vi "Scripting_GetNoErrorInsideTerminals.vi"(0 "ViReference":refnum<vi>, 5 "error in (no error)":errorcluster, 6 "RemoveWire(False)":bool, 7 "OnlyTop(False)":bool, 8 "GetCaseLeftTerminals(True)":bool=TRUE) -> (13 "Bottom_InsideTermRefnumOut":refnum<vi>, 14 "Top_WireTermSource":refnum<vi>, 15 "Top_WireTermDrains":refnum<vi>[](array[refnum]), 16 "Bottom_WireTermSource":refnum<vi>, 17 "Bottom_WireTermDrains":refnum<vi>[](array[refnum]), 18 "Top_InsideTermRefnumOut":refnum<vi>, 19 "error out":errorcluster)   [LabVIEW 2020]
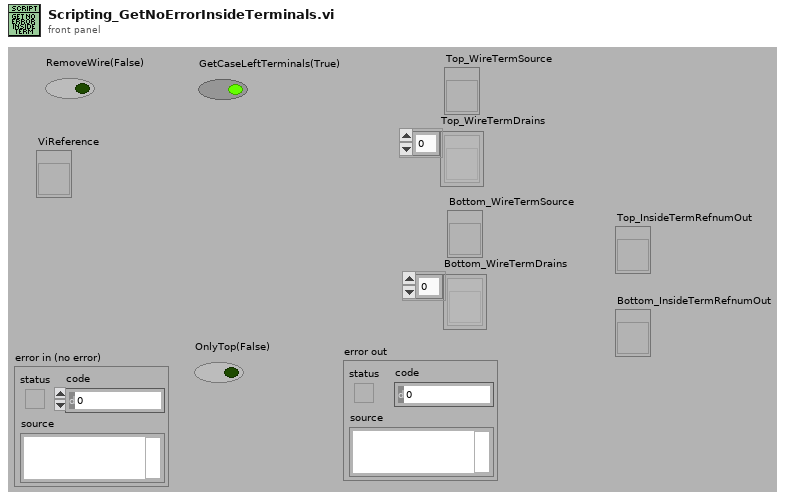
[diagram p1: front panel]
types:
  T1 = typedef "LVRectTypeDef.ctl" = cluster{"Left":i16, "Top":i16, "Right":i16, "Bottom":i16}
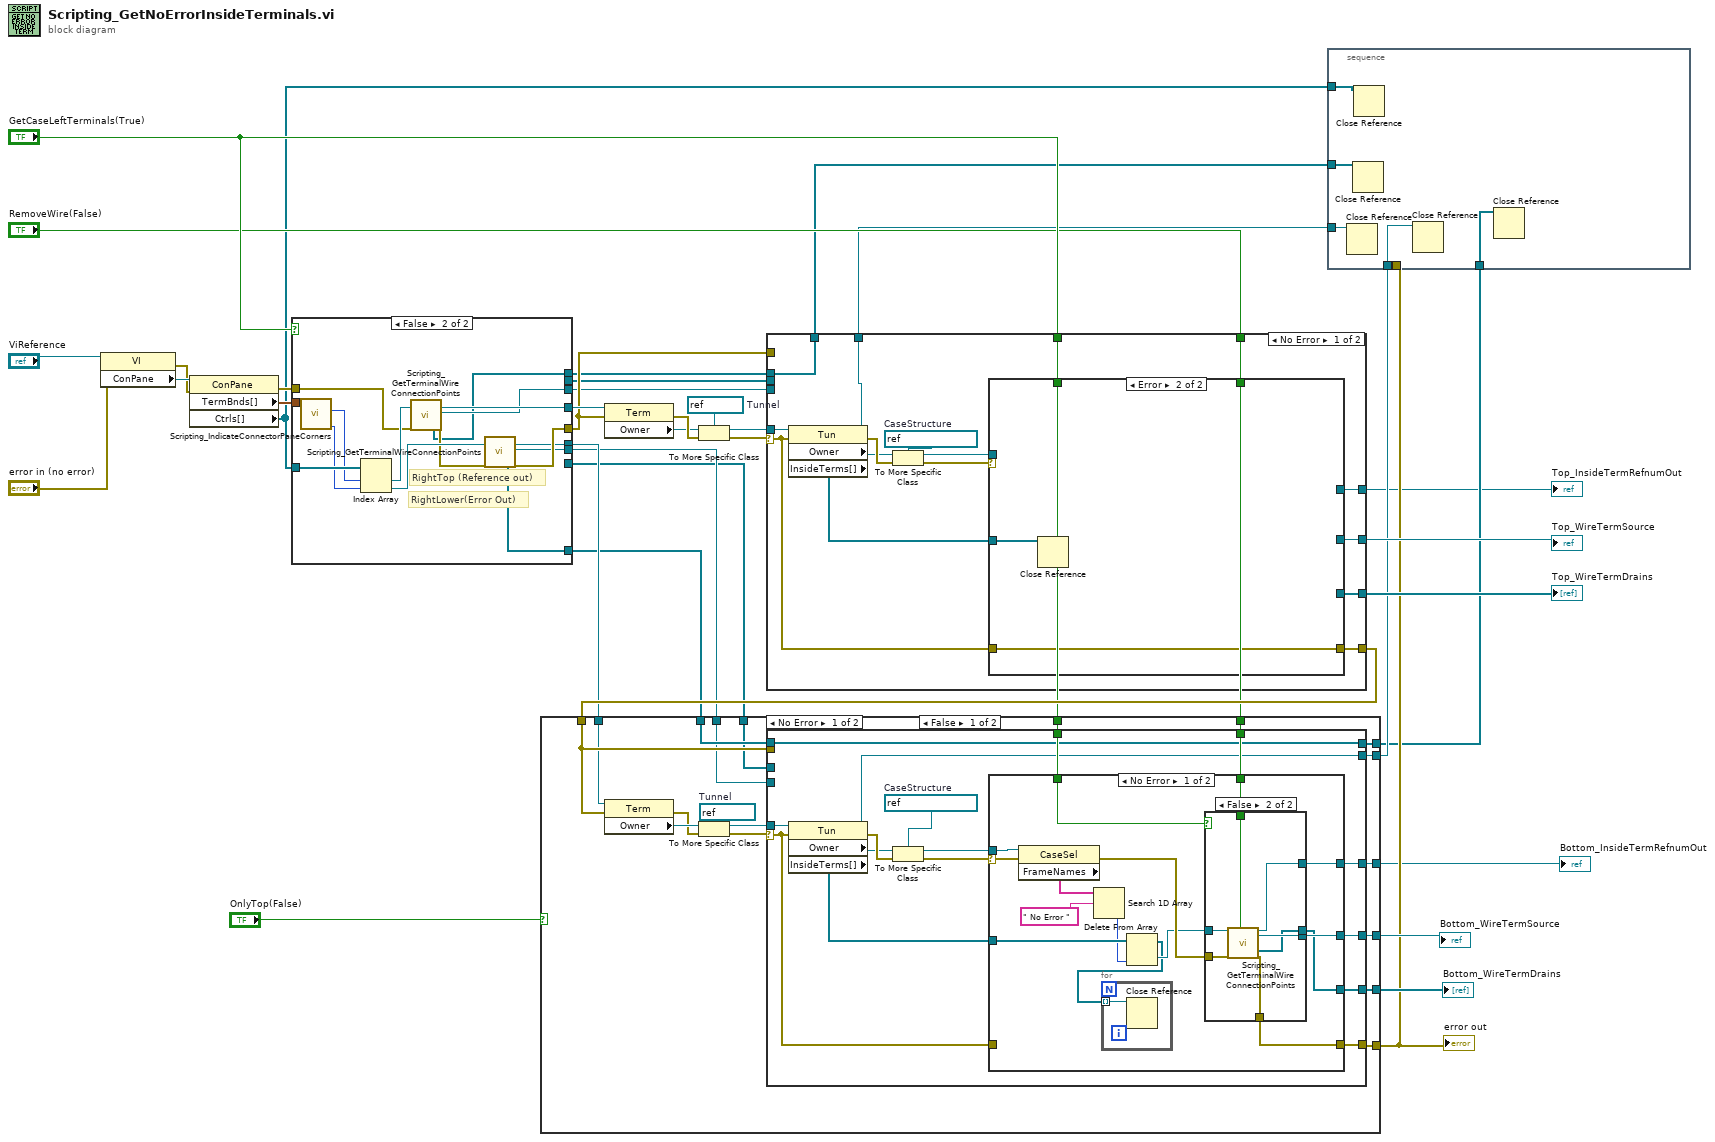
[diagram p0: block diagram]
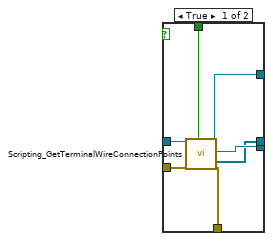
[diagram p2: hidden frame]
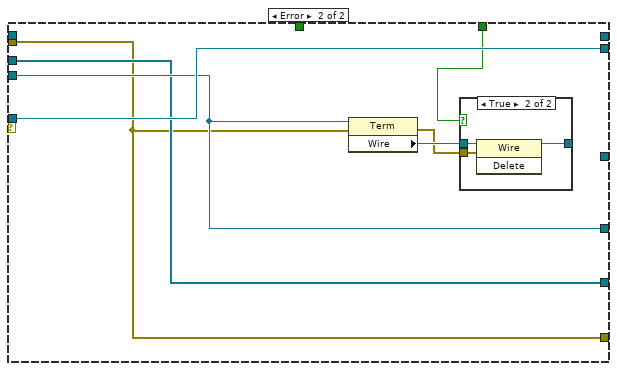
[diagram p4: hidden frame]
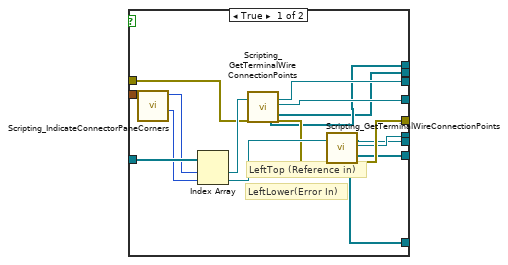
[diagram p7: hidden frame]
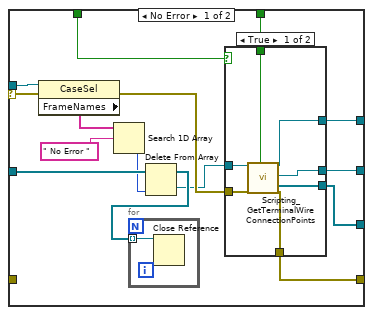
[diagram p8: hidden frame]
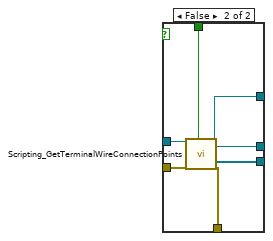
[diagram p9: hidden frame]
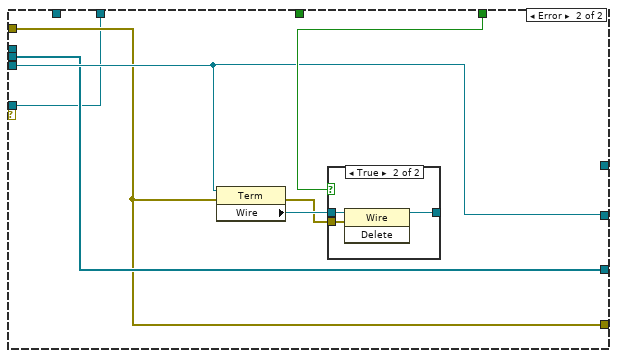
[diagram p10: hidden frame]
diagram:
  w32 = refnum<vi> refnum  # Tunnel
  n1 = property class="VI"(reference="ViReference", error in="error in (no error)") -> (error out=w23:errorcluster, "ConPane"=w35:refnum<vi>)  [unwired: 1 out]
  n2 = property class="ConPane"(reference=w35, error in=w23) -> (error out=w34:errorcluster, "TermBnds[]"=w36:T1[], "Ctrls[]"=w14:refnum<vi>[])  [unwired: 1 out]
  n3 = case shown="False" "GetCaseLeftTerminals(True)" {
    tunnel: w36 -> [w53 w68]
    tunnel: w14 -> [w52 w67]
    tunnel: w34 -> [w50 w63]
    tunnel: [w47 w62] -> w33
    tunnel: [w44 w59] -> w28
    tunnel: [w43 w58] -> w18
    tunnel: [w41 w55] -> w12
    tunnel: [w42 w57] -> w10
    tunnel: [w40 w56] -> w8
    tunnel: [w39 w54] -> w7
    tunnel: [w38 _] -> w5
    tunnel: [w37 _] -> w4
    frame True {
      # "LeftLower(Error In)"
      # "LeftTop (Reference in)"
      n4 = call "Scripting_IndicateConnectorPaneCorners.vi"("TermBnds[]"=w53) -> ("LeftLower"=w48:i32, "LeftTop"=w49:i32)  [unwired: 7 in, 2 out]
      n5 = Index Array(array=w52, index #1=w49, index #2=w48) -> (element #1=w51:refnum<vi>, element #2=w46:refnum<vi>)
      n6 = call "Scripting_GetTerminalWireConnectionPoints.vi"("ControlRef(IgnoredIfNotWired)"=w51, "error in"=w50) -> ("AllWireTerminals"=w41:refnum<vi>[], "WireTermSource"=w42:refnum<vi>, "FirstWireTermDrain"=w47:refnum<vi>, "AllWireTerminalDrains"=w37:refnum<vi>[], "error out"=w45:errorcluster)  [unwired: 9 in, 4 out]
      n7 = call "Scripting_GetTerminalWireConnectionPoints.vi"("ControlRef(IgnoredIfNotWired)"=w46, "error in"=w45) -> ("AllWireTerminals"=w40:refnum<vi>[], "WireTermSource"=w39:refnum<vi>, "FirstWireTermDrain"=w43:refnum<vi>, "AllWireTerminalDrains"=w38:refnum<vi>[], "error out"=w44:errorcluster)  [unwired: 9 in, 4 out]
    }
    frame False {
      # "RightLower(Error Out)"
      # "RightTop (Reference out)"
      n8 = call "Scripting_IndicateConnectorPaneCorners.vi"("TermBnds[]"=w68) -> ("RightLower"=w65:i32, "RightTop"=w66:i32)  [unwired: 7 in, 2 out]
      n9 = Index Array(array=w67, index #1=w66, index #2=w65) -> (element #1=w64:refnum<vi>, element #2=w61:refnum<vi>)
      n10 = call "Scripting_GetTerminalWireConnectionPoints.vi"("ControlRef(IgnoredIfNotWired)"=w64, "error in"=w63) -> ("AllWireTerminals"=w55:refnum<vi>[], "WireTermSource"=w62:refnum<vi>, "FirstWireTermDrain"=w57:refnum<vi>, "error out"=w60:errorcluster)  [unwired: 9 in, 5 out]
      n11 = call "Scripting_GetTerminalWireConnectionPoints.vi"("ControlRef(IgnoredIfNotWired)"=w61, "error in"=w60) -> ("AllWireTerminals"=w56:refnum<vi>[], "WireTermSource"=w58:refnum<vi>, "FirstWireTermDrain"=w54:refnum<vi>, "error out"=w59:errorcluster)  [unwired: 9 in, 5 out]
    }
  }
  n12 = property class="Term"(reference=w33, error in=w28) -> (error out=w31:errorcluster, "Owner"=w27:refnum<vi>)  [unwired: 1 out]
  n13 = To More Specific Class(target class=w32, reference=w27, error in=w31) -> (specific class reference=w29:refnum<vi>, error out=w30:errorcluster)
  n14 = case shown="No Error" w30 {
    selector: w30 -> [w75 _]
    tunnel: w29 -> [w84 w117]
    tunnel: w28 -> [_ w119]
    tunnel: [w78 w122] -> w26
    tunnel: [w77 w120] -> w25
    tunnel: [w76 w119] -> w21
    tunnel: "RemoveWire(False)" -> [w74 w123]
    tunnel: "GetCaseLeftTerminals(True)" -> [w72 _]
    tunnel: w12 -> [w71 _]
    tunnel: [w71 _] -> w11
    tunnel: w10 -> [_ w122]
    tunnel: w4 -> [_ w120]
    tunnel: [w70 w117] -> w3
    tunnel: [w69 _] -> w2
    frame No Error {
      w83 = refnum<vi> refnum  # CaseStructure
      n15 = property class="Tun"(reference=w84, error in=w75) -> (reference out=w70:refnum<vi>, error out=w80:errorcluster, "Owner"=w79:refnum<vi>, "InsideTerms[]"=w73:refnum<vi>[])
      n16 = To More Specific Class(target class=w83, reference=w79, error in=w80) -> (specific class reference=w82:refnum<vi>, error out=w81:errorcluster)
      n17 = case shown="Error" w81 {
        selector: w81 -> [w92 _]
        tunnel: w82 -> [w97 _]
        tunnel: [w95 _] -> w78
        tunnel: [w94 _] -> w77
        tunnel: [w93 w116] -> w76
        tunnel: w75 -> [_ w116]
        tunnel: w74 -> [w91 _]
        tunnel: w73 -> [w90 w115]
        tunnel: w72 -> [w88 _]
        tunnel: [w85 _] -> w69
        frame No Error {
          n18 = property class="CaseSel"(reference=w97, error in=w92) -> (error out=w96:errorcluster, "FrameNames"=w99:string[])  [unwired: 1 out]
          n19 = Search 1D Array(1D array=w99, element=" No Error ") -> (index of element=w89:i32)  [unwired: 1 in]
          n20 = Delete From Array(array=w90, index=w89) -> (deleted portion=w86:refnum<vi>, array with subset deleted=w87:refnum<vi>[])  [unwired: 1 in]
          n21 = for {
            tunnel: w87 -> [w100] mode=indexing
            n22 = Close Reference(reference=w100) -> ()  [unwired: 1 in, 1 out]
          }
          n23 = case shown="True" w88 {
            tunnel: w96 -> [w107 w114]
            tunnel: [w103 w113] -> w95
            tunnel: [w102 w109] -> w94
            tunnel: [w106 w112] -> w93
            tunnel: w91 -> [w105 w111]
            tunnel: w86 -> [w104 w110]
            tunnel: [w101 w108] -> w85
            frame True {
              n24 = call "Scripting_GetTerminalWireConnectionPoints.vi"("Term Refnum In"=w104, "error in"=w107, "RemoveWire(False)"=w105) -> ("Term Refnum Out"=w101:refnum<vi>, "FirstWireTermDrain"=w103:refnum<vi>, "AllWireTerminalDrains"=w102:refnum<vi>[], "error out"=w106:errorcluster)  [unwired: 8 in, 5 out]
            }
            frame False {
              n25 = call "Scripting_GetTerminalWireConnectionPoints.vi"("Term Refnum In"=w110, "error in"=w114, "RemoveWire(False)"=w111) -> ("Term Refnum Out"=w108:refnum<vi>, "WireTermSource"=w113:refnum<vi>, "AllWireTerminalDrains"=w109:refnum<vi>[], "error out"=w112:errorcluster)  [unwired: 8 in, 5 out]
            }
          }
        }
        frame Error {
          n26 = Close Reference(reference=w115) -> ()  [unwired: 1 in, 1 out]
        }
      }
    }
    frame Error {
      n27 = property class="Term"(reference=w122, error in=w119) -> (error out=w118:errorcluster, "Wire"=w121:refnum<vi>)  [unwired: 1 out]
      n28 = case shown="True" w123 {
        tunnel: [w124 w127] -> _
        tunnel: w121 -> [w124 w126]
        tunnel: w118 -> [_ w125]
        frame False {
        }
        frame True {
          n29 = invoke class="Wire" method="Delete"(reference=w126, error in=w125) -> (reference out=w127:refnum<vi>)  [unwired: 1 in, 2 out]
        }
      }
    }
  }
  "Top_WireTermSource" <- w26
  "Top_WireTermDrains" <- w25
  "Top_InsideTermRefnumOut" <- w2
  n30 = case shown="False" "OnlyTop(False)" {
    tunnel: w21 -> [w140 w205]
    tunnel: [w139 _] -> w20
    tunnel: [w138 _] -> w19
    tunnel: w18 -> [w137 _]
    tunnel: "GetCaseLeftTerminals(True)" -> [w136 _]
    tunnel: "RemoveWire(False)" -> [w135 _]
    tunnel: [w134 w205] -> w15
    tunnel: [w133 _] -> w13
    tunnel: [w132 w204] -> w9
    tunnel: w8 -> [w131 w204]
    tunnel: w7 -> [w130 _]
    tunnel: w5 -> [w129 _]
    tunnel: [w128 _] -> w1
    frame False {
      w141 = refnum<vi> refnum  # Tunnel
      n31 = property class="Term"(reference=w137, error in=w140) -> (error out=w142:errorcluster, "Owner"=w145:refnum<vi>)  [unwired: 1 out]
      n32 = To More Specific Class(target class=w141, reference=w145, error in=w142) -> (specific class reference=w144:refnum<vi>, error out=w143:errorcluster)
      n33 = case shown="No Error" w143 {
        selector: w143 -> [w152 _]
        tunnel: w144 -> [w161 w199]
        tunnel: w140 -> [_ w194]
        tunnel: [w155 w196] -> w139
        tunnel: [w154 w195] -> w138
        tunnel: [w153 w194] -> w134
        tunnel: w135 -> [w151 w197]
        tunnel: w136 -> [w149 _]
        tunnel: [w148 w199] -> w133
        tunnel: [w147 _] -> w132
        tunnel: w131 -> [w147 _]
        tunnel: w130 -> [_ w196]
        tunnel: w129 -> [_ w195]
        tunnel: [w146 _] -> w128
        frame No Error {
          w160 = refnum<vi> refnum  # CaseStructure
          n34 = property class="Tun"(reference=w161, error in=w152) -> (reference out=w148:refnum<vi>, error out=w157:errorcluster, "Owner"=w156:refnum<vi>, "InsideTerms[]"=w150:refnum<vi>[])
          n35 = To More Specific Class(target class=w160, reference=w156, error in=w157) -> (specific class reference=w159:refnum<vi>, error out=w158:errorcluster)
          n36 = case shown="No Error" w158 {
            selector: w158 -> [w169 _]
            tunnel: w159 -> [w174 _]
            tunnel: [w172 _] -> w155
            tunnel: [w171 _] -> w154
            tunnel: [w170 w192] -> w153
            tunnel: w152 -> [_ w192]
            tunnel: w151 -> [w168 _]
            tunnel: w150 -> [w166 _]
            tunnel: w149 -> [w167 _]
            tunnel: [w162 _] -> w146
            frame No Error {
              n37 = property class="CaseSel"(reference=w174, error in=w169) -> (error out=w173:errorcluster, "FrameNames"=w176:string[])  [unwired: 1 out]
              n38 = Search 1D Array(1D array=w176, element=" No Error ") -> (index of element=w165:i32)  [unwired: 1 in]
              n39 = Delete From Array(array=w166, index=w165) -> (deleted portion=w164:refnum<vi>, array with subset deleted=w163:refnum<vi>[])  [unwired: 1 in]
              n40 = for {
                tunnel: w163 -> [w177] mode=indexing
                n41 = Close Reference(reference=w177) -> ()  [unwired: 1 in, 1 out]
              }
              n42 = case shown="False" w167 {
                tunnel: w173 -> [w184 w191]
                tunnel: [w180 w190] -> w172
                tunnel: [w179 w186] -> w171
                tunnel: [w183 w189] -> w170
                tunnel: w168 -> [w182 w188]
                tunnel: w164 -> [w181 w187]
                tunnel: [w178 w185] -> w162
                frame True {
                  n43 = call "Scripting_GetTerminalWireConnectionPoints.vi"("Term Refnum In"=w181, "error in"=w184, "RemoveWire(False)"=w182) -> ("Term Refnum Out"=w178:refnum<vi>, "FirstWireTermDrain"=w180:refnum<vi>, "AllWireTerminalDrains"=w179:refnum<vi>[], "error out"=w183:errorcluster)  [unwired: 8 in, 5 out]
                }
                frame False {
                  n44 = call "Scripting_GetTerminalWireConnectionPoints.vi"("Term Refnum In"=w187, "error in"=w191, "RemoveWire(False)"=w188) -> ("Term Refnum Out"=w185:refnum<vi>, "WireTermSource"=w190:refnum<vi>, "AllWireTerminalDrains"=w186:refnum<vi>[], "error out"=w189:errorcluster)  [unwired: 8 in, 5 out]
                }
              }
            }
            frame Error {
            }
          }
        }
        frame Error {
          n45 = property class="Term"(reference=w196, error in=w194) -> (error out=w193:errorcluster, "Wire"=w198:refnum<vi>)  [unwired: 1 out]
          n46 = case shown="True" w197 {
            tunnel: [w200 w203] -> _
            tunnel: w198 -> [w200 w202]
            tunnel: w193 -> [_ w201]
            frame False {
            }
            frame True {
              n47 = invoke class="Wire" method="Delete"(reference=w202, error in=w201) -> (reference out=w203:refnum<vi>)  [unwired: 1 in, 2 out]
            }
          }
        }
      }
    }
    frame True {
    }
  }
  "error out" <- w15
  "Bottom_WireTermSource" <- w20
  "Bottom_WireTermDrains" <- w19
  "Bottom_InsideTermRefnumOut" <- w1
  n48 = stacked-sequence {
    tunnel: w15 -> [_]
    tunnel: w14 -> [w208]
    tunnel: w13 -> [w210]
    tunnel: w11 -> [w207]
    tunnel: w9 -> [w206]
    tunnel: w3 -> [w209]
    frame #0 {
      n49 = Close Reference(reference=w209) -> ()  [unwired: 1 in, 1 out]
      n50 = Close Reference(reference=w207) -> ()  [unwired: 1 in, 1 out]
      n51 = Close Reference(reference=w208) -> ()  [unwired: 1 in, 1 out]
      n52 = Close Reference(reference=w210) -> ()  [unwired: 1 in, 1 out]
      n53 = Close Reference(reference=w206) -> ()  [unwired: 1 in, 1 out]
    }
  }
